vi "PH_VacuumControl.prepare historical Data.vi"(7 "Start Fit":dbl, 8 "Limit":dbl, 9 "Timebase [s]":i32[](array[numeric]), 10 "Pressure [mbar]":dbl[](array[numeric])) -> (1 "Trend":cluster{i32[], "Data":dbl[]}[](graph), 2 "Time to reach Limit":dbl)   [LabVIEW 2014, in "PH_VacuumControl.lvlib"]
doc: "Within this VI the data are prepared for presentation at the GUI and a trend calculation is tried."
uses:
  PH_VacuumControl.lvlib
  <vilib>/Analysis/NI_AALPro.lvlib
panel:
  in  "parameter bounds":T1={"amp min"=-inf, "amp max"=inf, "damping min"=-inf, "damping max"=inf, "offset min"=0.0, "offset max"=0.0}
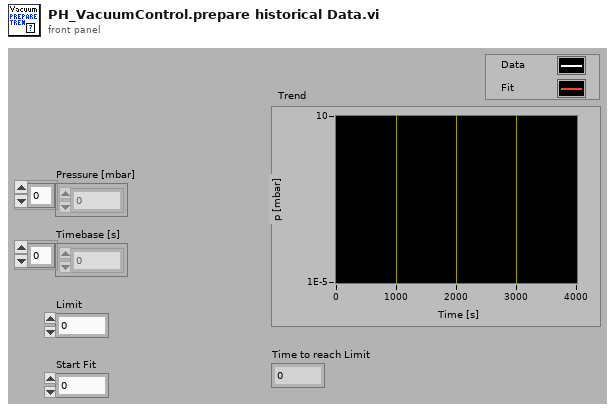
[diagram p1: front panel]
types:
  T1 = cluster{"amp min":dbl, "amp max":dbl, "damping min":dbl, "damping max":dbl, "offset min":dbl, "offset max":dbl}
  T2 = cluster{"Timebase [s]":i32[], "Pressure [mbar]":dbl[]}
  T3 = cluster{"Timebase [s]":i32[], "Best Exponential Fit":dbl[]}[]
  T4 = cluster{"Timebase [s]":i32[], "Pressure [mbar]":dbl[]}[]
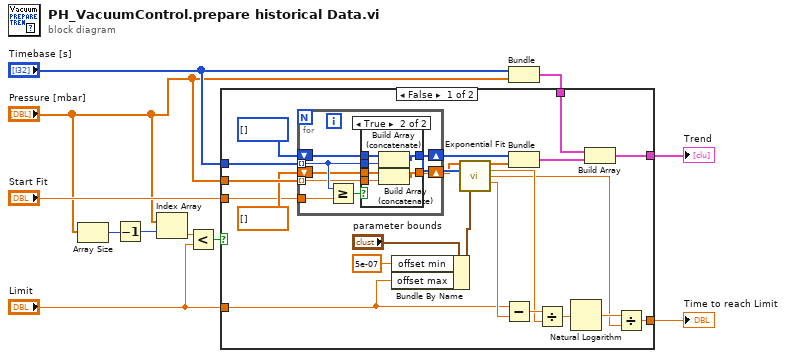
[diagram p0: block diagram]
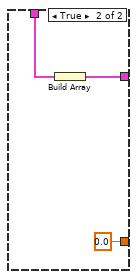
[diagram p3: hidden frame]
diagram:
  n1 = Array Size(array="Pressure [mbar]") -> (size(s)=w8:i32)
  n2 = Decrement(x=w8) -> (x-1=w6:i32)
  n3 = Index Array(array="Pressure [mbar]", index=w6) -> (element=w5:dbl)
  n4 = Less?(x=w5, y="Limit") -> (x < y?=w3:bool)
  n5 = Bundle("Timebase [s]"="Timebase [s]", "Pressure [mbar]"="Pressure [mbar]") -> (w1:T2)  [unwired: 1 in]
  n6 = case shown="False" w3 {
    tunnel: w1 -> [w12 w52]
    tunnel: [w26 0.0] -> w11
    tunnel: "Timebase [s]" -> [w22 _]
    tunnel: "Pressure [mbar]" -> [w21 _]
    tunnel: "Start Fit" -> [w16 _]
    tunnel: "Limit" -> [w15 _]
    tunnel: [w13 w51] -> w2
    frame False {
      n7 = for {
        tunnel: w22 -> [w39] mode=indexing
        tunnel: w21 -> [w34] mode=indexing
        tunnel: w16 -> [w41]
        shift-right: [w38] -> w20
        shift-left: i32[] [] -> [w37]
        shift-right: [w36] -> w19
        shift-left: dbl[] [] -> [w35]
        n8 = Greater Or Equal?(x=w39, y=w41) -> (x >= y?=w40:bool)
        n9 = case shown="True" w40 {
          tunnel: w39 -> [_ w49]
          tunnel: [w43 w48] -> w38
          tunnel: w37 -> [w43 w47]
          tunnel: [w42 w46] -> w36
          tunnel: w35 -> [w42 w45]
          tunnel: w34 -> [_ w44]
          frame False {
          }
          frame True {
            n10 = Build Array (concatenate)(w47, w49) -> (w48:i32[])
            n11 = Build Array (concatenate)(w45, w44) -> (w46:dbl[])
          }
        }
      }
      n12 = Bundle By Name(cluster="parameter bounds", "offset min"=5e-07, "offset max"=w15) -> (w24:T1)
      n13 = call <vilib>:"Exponential Fit.vi"("Y"=w19, "X"=w20, "parameter bounds"=w24) -> ("Best Exponential Fit"=w33:dbl[], "amplitude"=w30:dbl, "damping"=w27:dbl, "offset"=w32:dbl)  [unwired: 7 in, 2 out]
      n14 = Subtract(x=w15, y=w32) -> (x-y=w31:dbl)
      n15 = Bundle(w20, "Best Exponential Fit"=w33) -> (w14:cluster{i32[], "Best Exponential Fit":dbl[]})  [unwired: 1 in]
      n16 = Divide(x=w31, y=w30) -> (x/y=w29:dbl)
      n17 = Natural Logarithm(1:w29) -> (0:w28:dbl)
      n18 = Build Array(w12, w14) -> (w13:T3)
      n19 = Divide(x=w28, y=w27) -> (x/y=w26:dbl)
    }
    frame True {
      n20 = Build Array(w52) -> (w51:T4)
    }
  }
  "Trend" <- w2
  "Time to reach Limit" <- w11
